vi "FILE READ FROM CSV.vi"(0 "File Path":string="C:\\data\\07_34_08_PM_01_July_2026\\07_34_08_PM_01_July_202607_34_08_PM_01_July_2026.csv", 5 "X-AXIS":u16(ring) items=["None", "Time ( Sec )", "Normal Load ( N )", "Frictional Force ( N )", "Coefficient of Friction", "Depth ( Microns )", "Speed ( RPM )", "Frequency ( Hz )", "Angle ( Degree )", "Cyclic Friction Force ( N )", "Cyclic Co efficient Friction ", "Stage temperature ( Degree celcius )", "Sample temperature ( Degree celcius )", "Stroke Length ( mm )", "Scratch Speed ( mm/sec )", "Amb Humidity ( % Rh ) ", "Amb Temperature (Deg C)", "Acoustic (mV)", "Mx (Nm)", "My (Nm)", "Mz (Nm)", "Humidity ( % Rh )", "Sliding Distance (mm)", "Wear Track Diameter (mm)", "Fx(N)", "Fy(N)", "MTM BallSpeed (RPM)", "MTM DiscSpeed (RPM)", "Entrainment Speed", "Slide Role", "Slip(%)", "Rotary Speed (m/sec)", "MTM Ball Speed (m/sec)", "MTM Disc Speed (m/sec)", "ECR (ohms)"], 9 "Y-AXIS":u16(ring) items=["None", "Time ( Sec )", "Normal Load ( N )", "Frictional Force ( N )", "Coefficient of Friction", "Depth ( Microns )", "Speed ( RPM )", "Frequency ( Hz )", "Angle ( Degree )", "Cyclic Friction Force ( N )", "Cyclic Co efficient Friction ", "Stage temperature ( Degree celcius )", "Sample temperature ( Degree celcius )", "Stroke Length ( mm )", "Scratch Speed ( mm/sec )", "Amb Humidity ( % Rh ) ", "Amb Temperature (Deg C)", "Acoustic (mV)", "Mx (Nm)", "My (Nm)", "Mz (Nm)", "Humidity ( % Rh )", "Sliding Distance (mm)", "Wear Track Diameter (mm)", "Fx(N)", "Fy(N)", "MTM BallSpeed (RPM)", "MTM DiscSpeed (RPM)", "Entrainment Speed", "Slide Role", "Slip(%)", "Rotary Speed (m/sec)", "MTM Ball Speed (m/sec)", "MTM Disc Speed (m/sec)", "ECR (ohms)"], 11 "error in (no error)":errorcluster) -> (4 "output cluster":cluster{"X":dbl[], "Y":dbl[]}, 6 "mean":dbl format="%0.2f", 8 "standard deviation":dbl format="%0.2f", 10 "variance":dbl format="%0.2f", 15 "error out":errorcluster)   [LabVIEW 2025]
uses:
  <vilib>/Utility/file.llb/Read Delimited Spreadsheet (DBL).vi
  <vilib>/Analysis/NI_AALBase.lvlib
panel:
  # "C:\\data\\07_34_08_PM_01_July_2026\\07_34_08_PM_01_July_202607_34_08_PM_01_July_2026.csv"
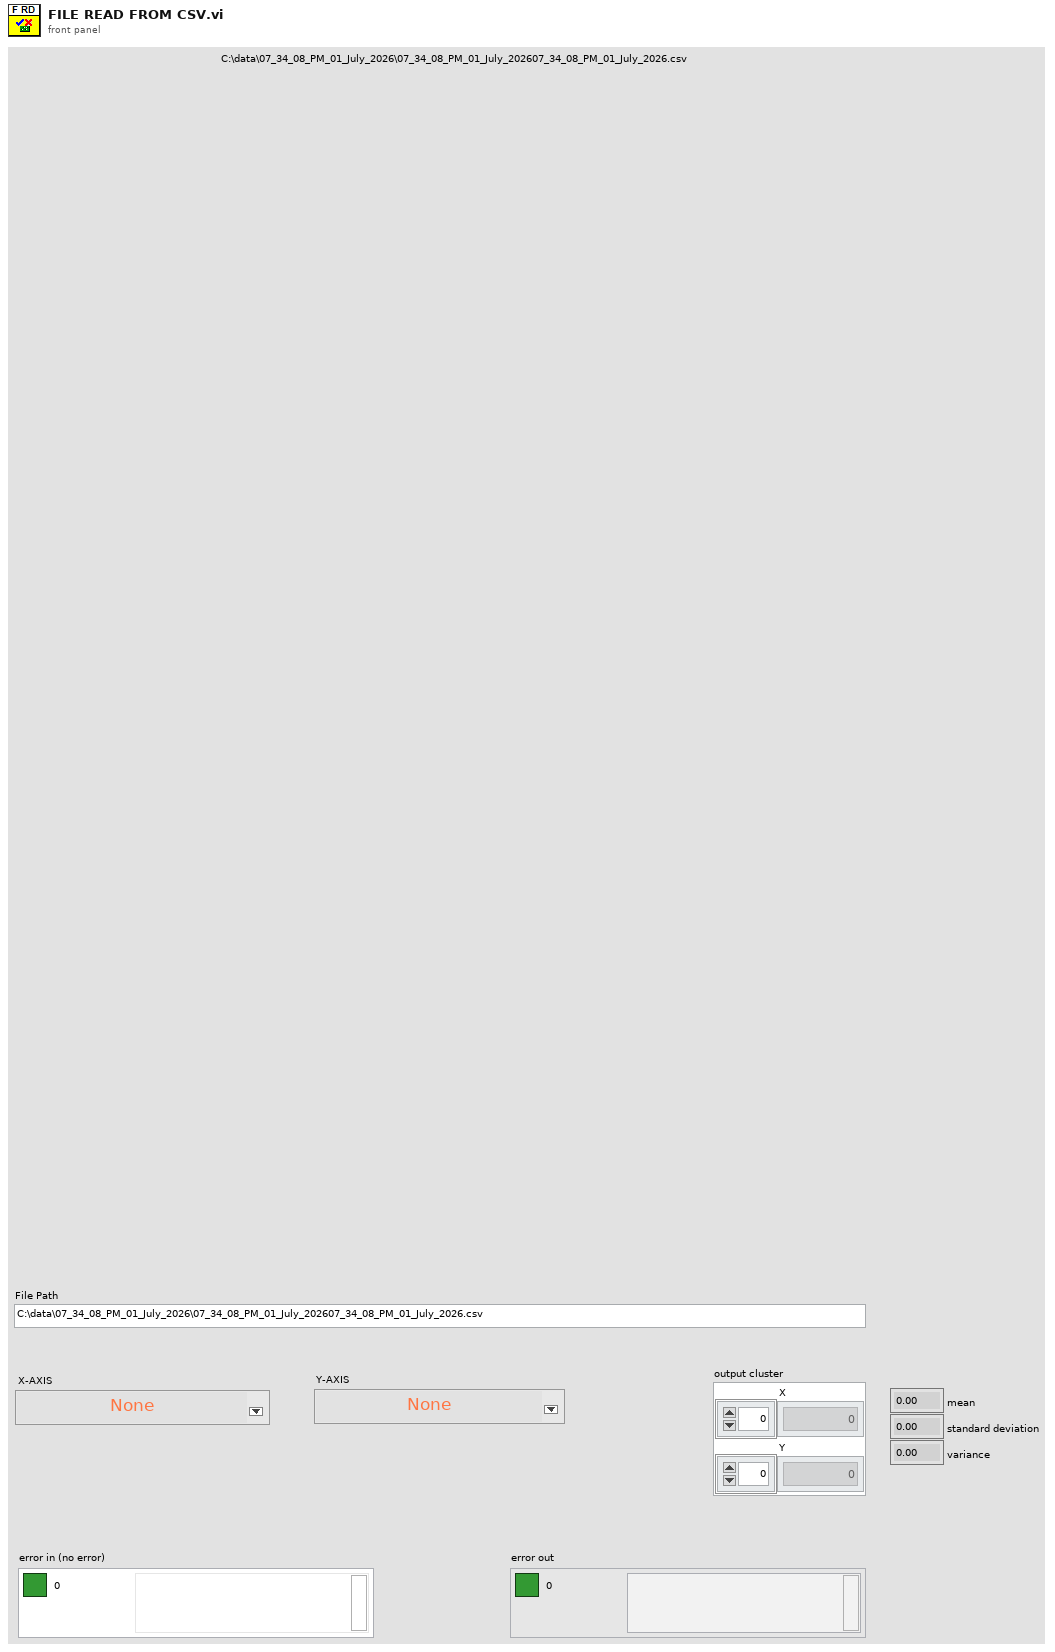
[diagram p1: front panel]
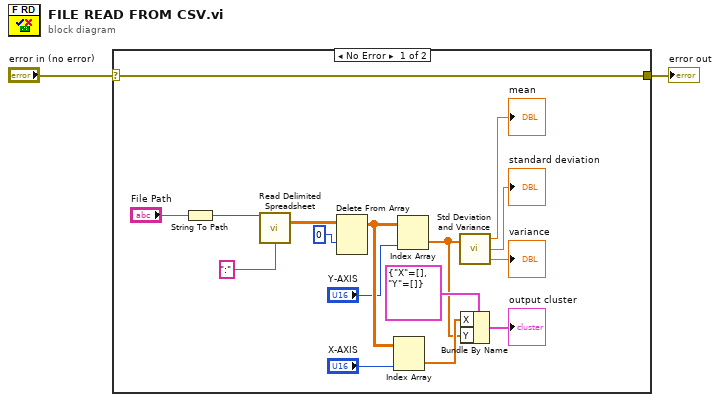
[diagram p0: block diagram]
diagram:
  n1 = case shown="No Error" "error in (no error)" {
    selector: "error in (no error)" -> [w7 _]
    tunnel: [w7 _] -> w1
    frame No Error {
      n2 = String To Path(string="File Path") -> (path=w17:path)
      n3 = call-poly <vilib>:"Read Delimited Spreadsheet.vi"("file path (dialog if empty)"=w17, "delimiter (\\t)"=":" ("delimiter (\\t)")) -> ("all rows"=w15:dbl[][])  [unwired: 8 in, 5 out]
      n4 = Delete From Array(array=w15, index (row)=0) -> (array with subset deleted=w12:dbl[][])  [unwired: 2 in, 1 out]
      n5 = Index Array(array=w12, index (col)="X-AXIS") -> (element=w9:dbl[])  [unwired: 1 in]
      n6 = Index Array(array=w12, index (col)="Y-AXIS") -> (element=w6:dbl[])  [unwired: 1 in]
      n7 = call <vilib>:"Std Deviation and Variance.vi"("X"=w6) -> ("mean"=→"mean":dbl, "standard deviation"=→"standard deviation":dbl, "variance"=→"variance":dbl)  [unwired: 1 in]
      n8 = Bundle By Name(cluster=cluster{"X":dbl[], "Y":dbl[]} {"X"=[], "Y"=[]} ("new element/subarray"), "X"=w9, "Y"=w6) -> (→"output cluster":cluster{"X":dbl[], "Y":dbl[]})
    }
    frame Error {
    }
  }
  "error out" <- w1
